vi "Sistema_Aquisicao_queued.vi"() -> ()   [LabVIEW 2012]
uses:
  Global_Telescopio.vi
panel:
  out "respQ":refnum<queue>
  out "cmdQ":refnum<queue>
  out "error out":errorcluster
  out "ultimo valor 2":dbl format="%#_9g"
  out "ultimo valor":dbl format="%#_9g"
  out "ultimo comando":dbl
  in  "Case Constant\n(See Context Help)":bool=TRUE
  out "O Recebido":bool
  out "TimeoutAq":u32
  out "concatenated string":string
  out "Maq Satus":i32
  out "TX":string
  out "Data rx Aquisição":string
  # "2"
  # "R -->Registra Centragem\nS -->Status\nO -->OffSet\nF ---> Foco"
  # "3"
  # "4"
  # "5"
  # "!"
  # "!"
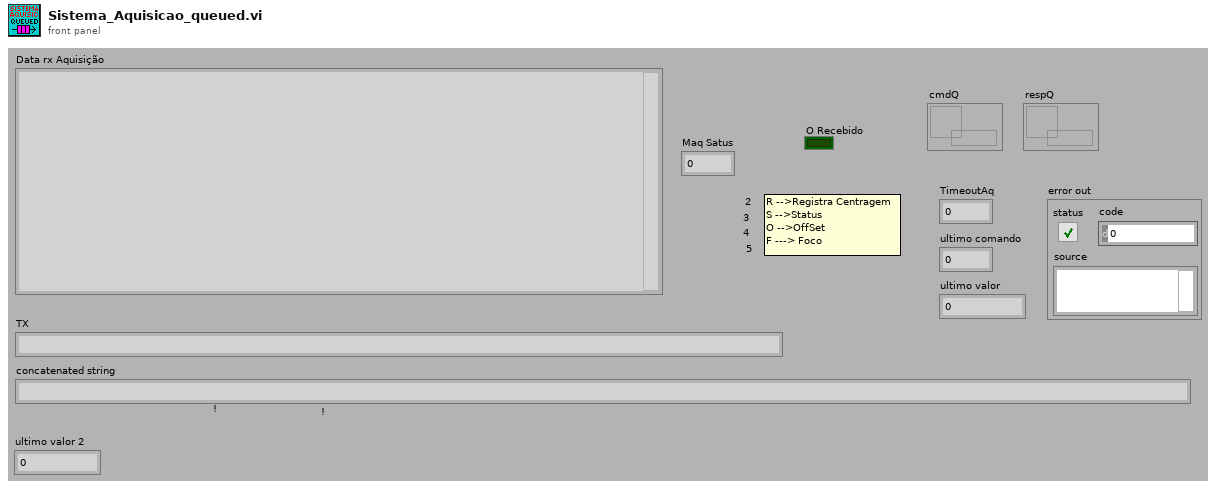
[diagram p1: front panel]
types:
  T1 = enum16{"open", "open or create", "create or replace", "create"}
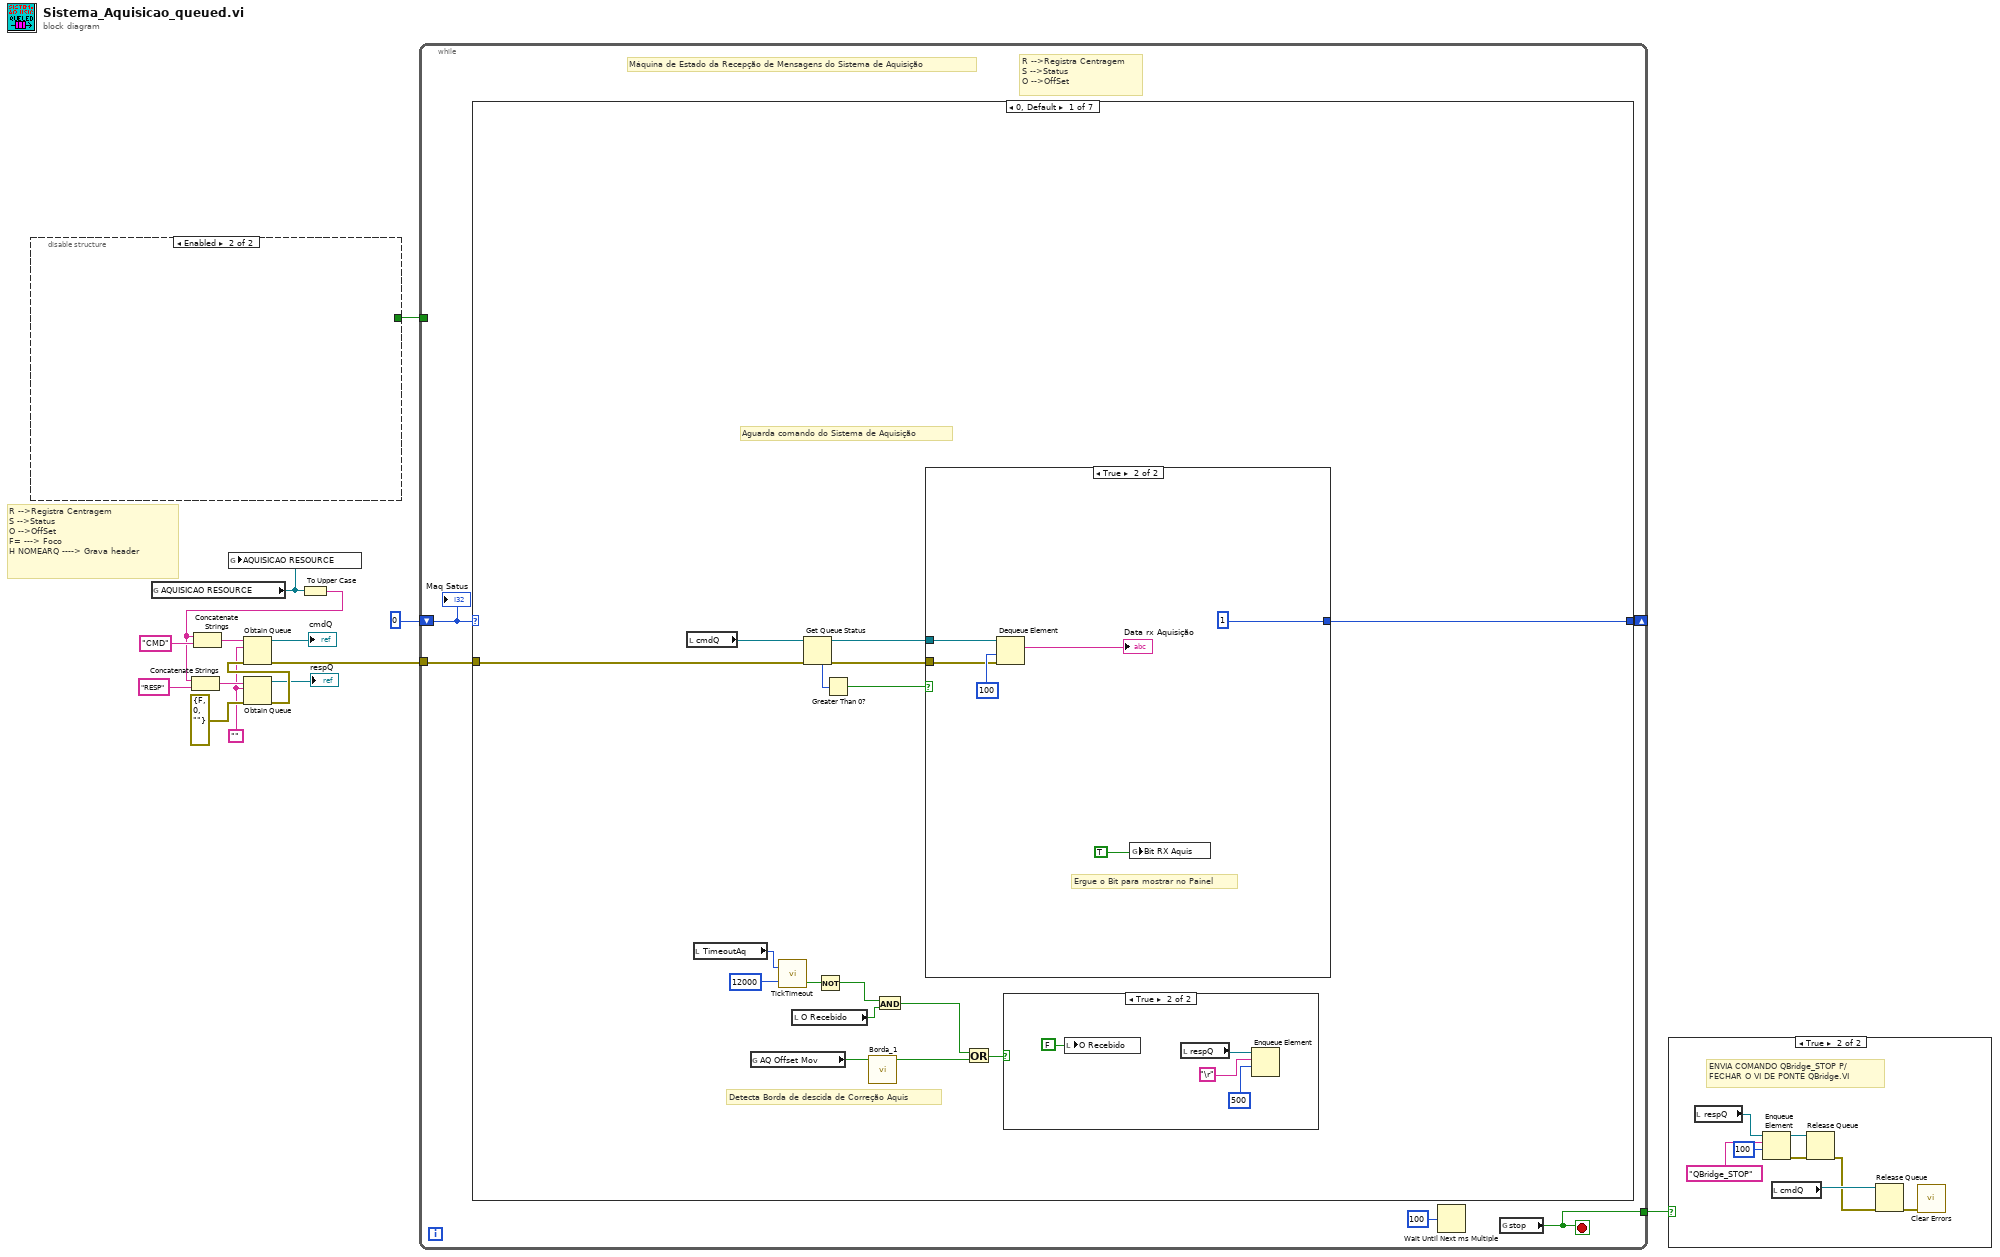
[diagram p0: block diagram]
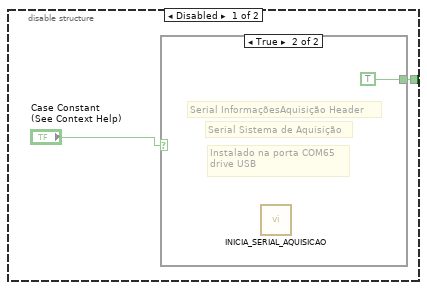
[diagram p3: hidden frame]
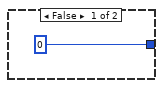
[diagram p6: hidden frame]
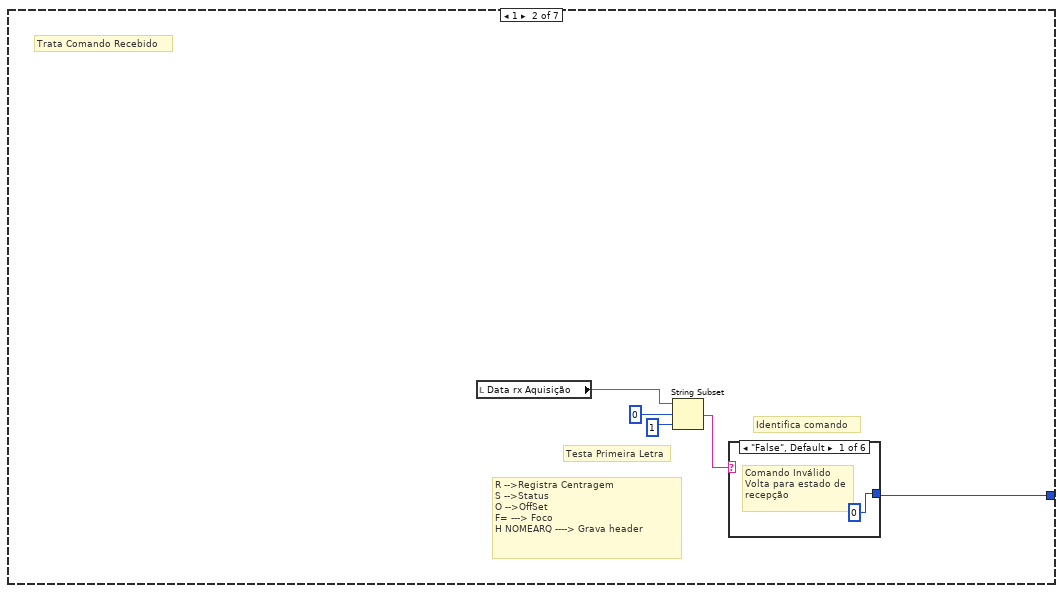
[diagram p7: hidden frame]
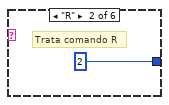
[diagram p8: hidden frame]
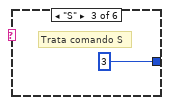
[diagram p9: hidden frame]
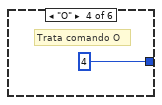
[diagram p10: hidden frame]
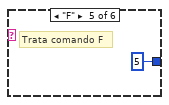
[diagram p11: hidden frame]
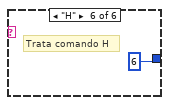
[diagram p12: hidden frame]
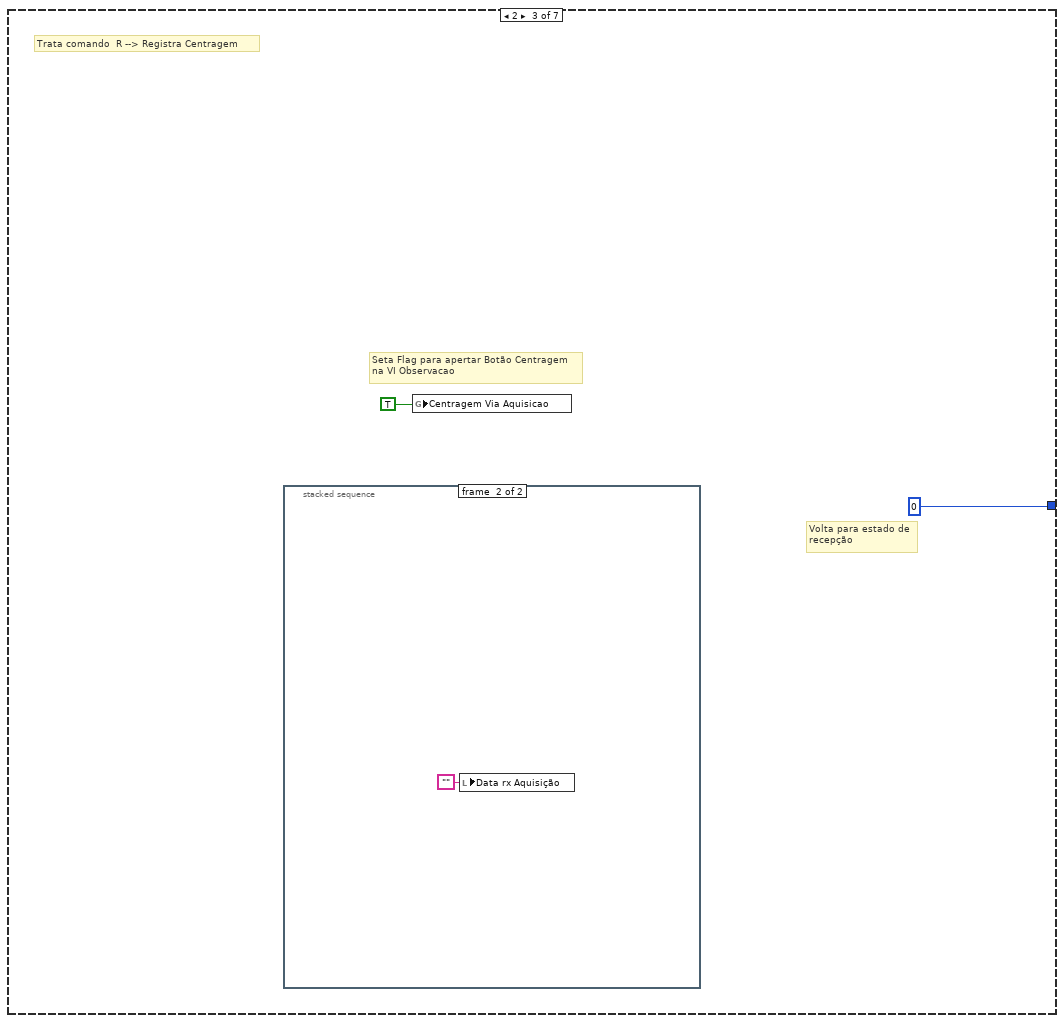
[diagram p13: hidden frame]
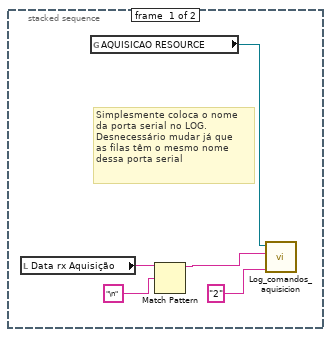
[diagram p14: hidden frame]
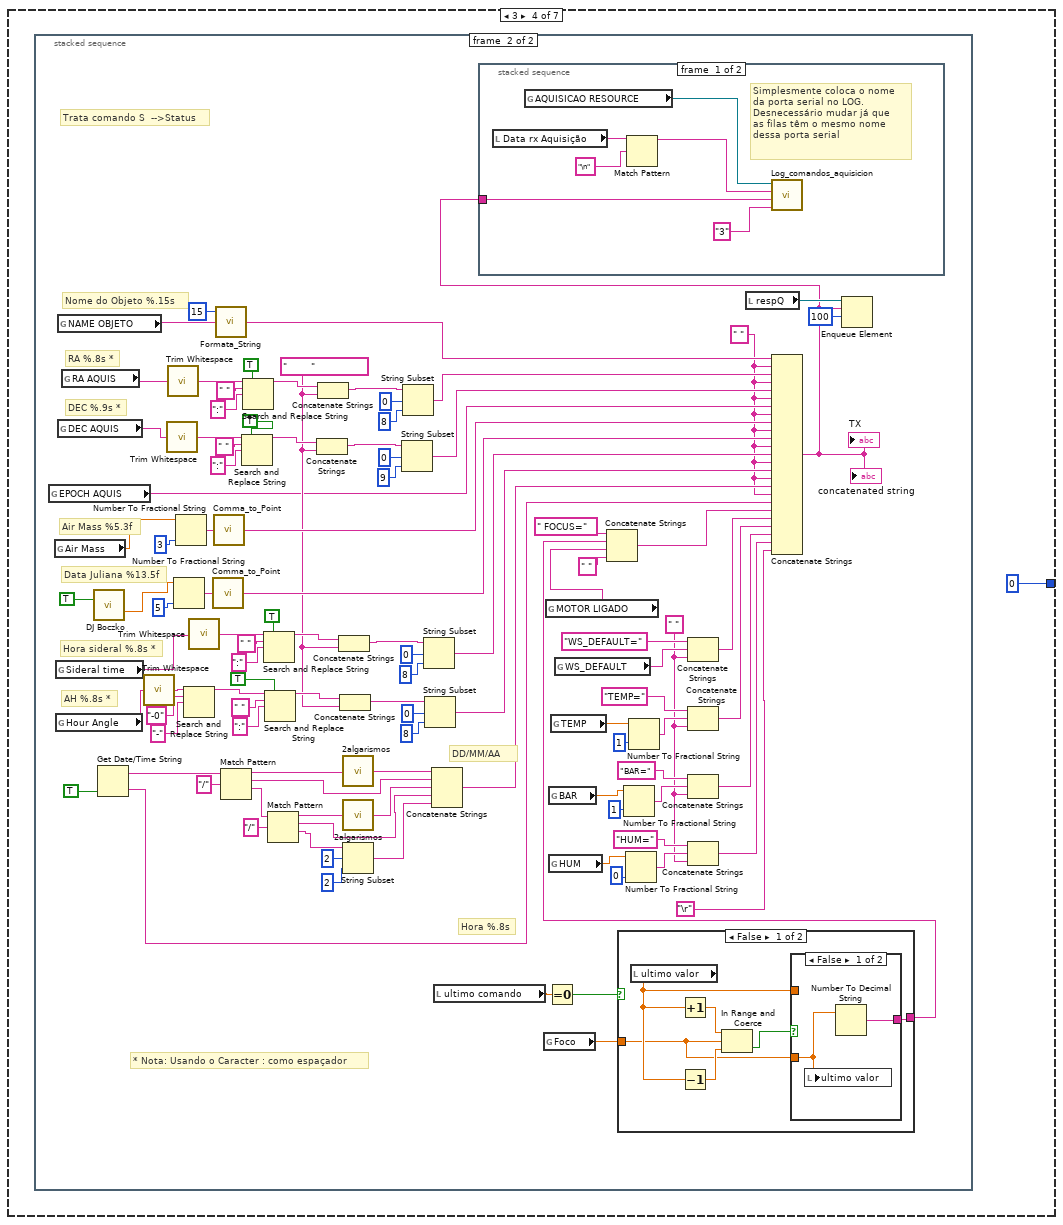
[diagram p15: hidden frame]
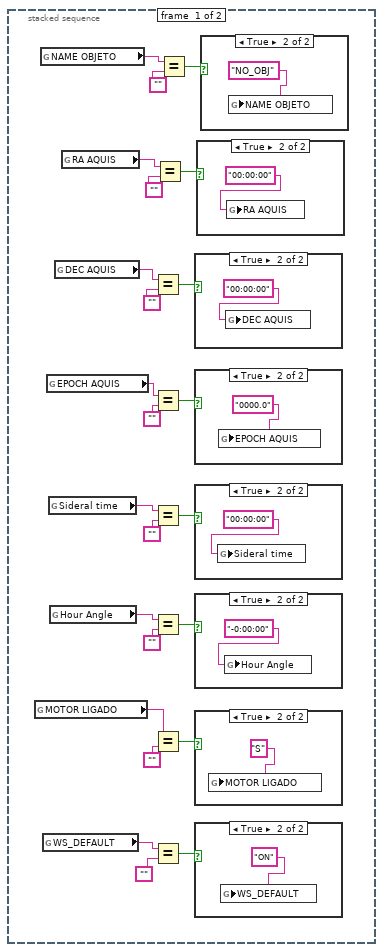
[diagram p16: hidden frame]
diagram:
  w5 = ""
  # "R -->Registra Centragem\nS -->Status\nO -->OffSet\nF= ---> Foco\nH NOMEARQ ----> Grava header"
  n1 = disable-structure shown="Enabled" {
    disable-tunnel: [w16 _] -> w14
    frame Disabled {
      n2 = case shown="True" "Case Constant\n(See Context Help)" {
        tunnel: [_ TRUE] -> w16
        frame False {
        }
        frame True {
          # "Instalado na porta COM65\ndrive USB"
          # "Serial Sistema de Aquisição"
          # "Serial InformaçõesAquisição Header"
          n3 = call "INICIA_SERIAL_AQUISICAO.vi"() -> ()  [unwired: 1 in]
        }
      }
    }
    frame Enabled {
    }
  }
  n4 = global read "Global_Telescopio.vi" "AQUISICAO RESOURCE"() -> (w3:refnum<visa-resource-name>)
  n5 = global write "Global_Telescopio.vi" "AQUISICAO RESOURCE"(w3) -> ()
  n6 = To Upper Case(1:w3) -> (0:w2:string)
  n7 = Concatenate Strings(w2, "RESP" ("string")) -> (w11:string)
  n8 = Concatenate Strings(w2, "CMD" ("string")) -> (w10:string)
  n9 = Obtain Queue(name (unnamed)=w11, element data type=w5, error in (no error)=errorcluster {"status"=FALSE, "code"=0, "source"=""}) -> (queue out=→"respQ":refnum<queue>, error out=w8:errorcluster)  [unwired: 2 in, 1 out]
  n10 = Obtain Queue(name (unnamed)=w10, element data type=w5, error in (no error)=w8) -> (queue out=→"cmdQ":refnum<queue>, error out=w4:errorcluster)  [unwired: 2 in, 1 out]
  n11 = while {
    shift-right: [w21] -> _
    shift-left: 0 -> [w22]
    tunnel: w14 -> [_]
    tunnel: w4 -> [w20]
    tunnel: [w19] -> w1
    stop <- w19 stop-if-true
    # "R -->Registra Centragem\nS -->Status\nO -->OffSet"
    # "Máquina de Estado da Recepção de Mensagens do Sistema de Aquisição"
    n12 = case shown="0, Default" w22 {
      tunnel: [w39 w51 0 0 0 0 0] -> w21
      tunnel: w20 -> [w25 _ _ _ _ _ _]
      frame 0, Default {
        # "Detecta Borda de descida de Correção Aquis"
        # "Aguarda comando do Sistema de Aquisição"
        n13 = local read "cmdQ"() -> (w24:refnum<queue>)
        n14 = local read "TimeoutAq"() -> (w32:u32)
        n15 = global read "Global_Telescopio.vi" "AQ Offset Mov"() -> (w37:bool)
        n16 = call "TickTimeout.vi"("msInicial"=w32, "msTimeout"=u32 12000) -> ("Timeout"=w33:bool)  [unwired: 2 out]
        n17 = local read "O Recebido"() -> (w35:bool)
        n18 = Get Queue Status(queue=w24, error in (no error)=w25) -> (queue out=w26:refnum<queue>, error out=w27:errorcluster, # elements in queue=w29:i32)  [unwired: 1 in, 5 out]
        n19 = Not(x=w33) -> (.not. x?=w31:bool)
        n20 = Greater Than 0?(x=w29) -> (x > 0?=w28:bool)
        n21 = call "Borda_1.vi"("Entrada"=w37) -> ("Boolean"=w38:bool)  [unwired: 4 in]
        n22 = And(x=w31, y=w35) -> (x .and. y?=w30:bool)
        n23 = case shown="True" w28 {
          tunnel: [0 1] -> w39
          tunnel: w27 -> [_ w46]
          tunnel: w26 -> [_ w47]
          frame False {
          }
          frame True {
            # "Ergue o Bit para mostrar no Painel"
            n24 = Dequeue Element(queue=w47, timeout in ms (-1)=100, error in (no error)=w46) -> (element=→"Data rx Aquisição":string)  [unwired: 3 out]
            n25 = global write "Global_Telescopio.vi" "Bit RX Aquis"(TRUE) -> ()
          }
        }
        n26 = Or(x=w30, y=w38) -> (x .or. y?=w36:bool)
        n27 = case shown="True" w36 {
          frame False {
          }
          frame True {
            n28 = local write "O Recebido"(FALSE ("O Recebido")) -> ()
            n29 = local read "respQ"() -> (w42:refnum<queue>)
            n30 = Enqueue Element(queue=w42, element="\r", timeout in ms (-1)=500) -> ()  [unwired: 1 in, 3 out]
          }
        }
      }
      frame 1 {
        # "R -->Registra Centragem\nS -->Status\nO -->OffSet\nF= ---> Foco\nH NOMEARQ ----> Grava header"
        # "Testa Primeira Letra"
        # "Identifica comando"
        # "Trata Comando Recebido"
        n31 = local read "Data rx Aquisição"() -> (w52:string)
        n32 = String Subset(string=w52, offset (0)=0, length (rest)=1 ("length (rest)")) -> (substring=w55:string)
        n33 = case shown="\"False\", Default" w55 {
          tunnel: [0 2 3 4 5 6] -> w51
          frame "False", Default {
            # "Comando Inválido\nVolta para estado de\nrecepção"
          }
          frame "R" {
            # "Trata comando R"
          }
          frame "S" {
            # "Trata comando S"
          }
          frame "O" {
            # "Trata comando O"
          }
          frame "F" {
            # "Trata comando F"
          }
          frame "H" {
            # "Trata comando H"
          }
        }
      }
      frame 2 {
        # "Seta Flag para apertar Botão Centragem\nna VI Observacao"
        # "Trata comando  R --> Registra Centragem"
        # "Volta para estado de\nrecepção"
        n34 = stacked-sequence {
          frame #0 {
            # "Simplesmente coloca o nome\nda porta serial no LOG.\nDesnecessário mudar já que \nas filas têm o mesmo nome\ndessa porta serial"
            n35 = local read "Data rx Aquisição"() -> (w65:string)
            n36 = global read "Global_Telescopio.vi" "AQUISICAO RESOURCE"() -> (w68:refnum<visa-resource-name>)
            n37 = Match Pattern(string=w65, regular expression="\n") -> (before substring=w64:string)  [unwired: 1 in, 3 out]
            n38 = call "Log_comandos_aquisicion.vi"("Estado"="2", "string de comando"=w64, "Porta"=w68) -> ()  [unwired: 9 in]
          }
          frame #1 {
            n39 = local write "Data rx Aquisição"("") -> ()
          }
        }
        n40 = global write "Global_Telescopio.vi" "Centragem Via Aquisicao"(TRUE ("Comunicaçao ok guider")) -> ()
      }
      frame 3 {
        n41 = stacked-sequence {
          frame #0 {
            n42 = global read "Global_Telescopio.vi" "MOTOR LIGADO"() -> (w91:string)
            n43 = global read "Global_Telescopio.vi" "NAME OBJETO"() -> (w72:string)
            n44 = global read "Global_Telescopio.vi" "WS_DEFAULT"() -> (w93:string)
            n45 = global read "Global_Telescopio.vi" "EPOCH AQUIS"() -> (w81:string)
            n46 = global read "Global_Telescopio.vi" "Sideral time"() -> (w83:string)
            n47 = global read "Global_Telescopio.vi" "Hour Angle"() -> (w88:string)
            n48 = global read "Global_Telescopio.vi" "DEC AQUIS"() -> (w79:string)
            n49 = global read "Global_Telescopio.vi" "RA AQUIS"() -> (w76:string)
            n50 = Equal?(x=w79, y="") -> (x = y?=w78:bool)
            n51 = Equal?(x=w81, y="") -> (x = y?=w80:bool)
            n52 = Equal?(x=w83, y="") -> (x = y?=w82:bool)
            n53 = Equal?(x=w88, y="") -> (x = y?=w84:bool)
            n54 = Equal?(x=w91, y="") -> (x = y?=w90:bool)
            n55 = Equal?(x=w93, y="") -> (x = y?=w92:bool)
            n56 = Equal?(x=w76, y="") -> (x = y?=w74:bool)
            n57 = Equal?(x=w72, y="") -> (x = y?=w73:bool)
            n58 = case shown="True" w78 {
              frame False {
              }
              frame True {
                n59 = global write "Global_Telescopio.vi" "DEC AQUIS"("00:00:00" ("NAME OBJETO")) -> ()
              }
            }
            n60 = case shown="True" w80 {
              frame False {
              }
              frame True {
                n61 = global write "Global_Telescopio.vi" "EPOCH AQUIS"("0000.0" ("NAME OBJETO")) -> ()
              }
            }
            n62 = case shown="True" w82 {
              frame False {
              }
              frame True {
                n63 = global write "Global_Telescopio.vi" "Sideral time"("00:00:00" ("NAME OBJETO")) -> ()
              }
            }
            n64 = case shown="True" w84 {
              frame False {
              }
              frame True {
                n65 = global write "Global_Telescopio.vi" "Hour Angle"("-0:00:00" ("NAME OBJETO")) -> ()
              }
            }
            n66 = case shown="True" w90 {
              frame False {
              }
              frame True {
                n67 = global write "Global_Telescopio.vi" "MOTOR LIGADO"("S") -> ()
              }
            }
            n68 = case shown="True" w92 {
              frame False {
              }
              frame True {
                n69 = global write "Global_Telescopio.vi" "WS_DEFAULT"("ON" ("Hora a ser Procurada")) -> ()
              }
            }
            n70 = case shown="True" w74 {
              frame False {
              }
              frame True {
                n71 = global write "Global_Telescopio.vi" "RA AQUIS"("00:00:00" ("NAME OBJETO")) -> ()
              }
            }
            n72 = case shown="True" w73 {
              frame False {
              }
              frame True {
                n73 = global write "Global_Telescopio.vi" "NAME OBJETO"("NO_OBJ" ("NAME OBJETO")) -> ()
              }
            }
          }
          frame #1 {
            w111 = " " ("string")
            w165 = "        " ("string")
            w120 = " "
            # "* Nota: Usando o Caracter : como espaçador"
            # "Hora %.8s"
            # "DD/MM/AA"
            # "AH %.8s *"
            # "Hora sideral %.8s *"
            # "Data Juliana %13.5f"
            # "Air Mass %5.3f"
            # "DEC %.9s *"
            # "RA %.8s *"
            # "Nome do Objeto %.15s"
            # "Trata comando S  -->Status"
            n74 = global read "Global_Telescopio.vi" "EPOCH AQUIS"() -> (w135:string)
            n75 = global read "Global_Telescopio.vi" "Air Mass"() -> (w144:dbl)
            n76 = global read "Global_Telescopio.vi" "Sideral time"() -> (w174:string)
            n77 = global read "Global_Telescopio.vi" "Hour Angle"() -> (w136:string)
            n78 = global read "Global_Telescopio.vi" "NAME OBJETO"() -> (w143:string)
            n79 = global read "Global_Telescopio.vi" "DEC AQUIS"() -> (w191:string)
            n80 = global read "Global_Telescopio.vi" "RA AQUIS"() -> (w206:string)
            n81 = call "DJ Boczko.vi"("TRUE = Hora Local\nFALSE = UT"=TRUE ("TRUE = Hora Local\nFALSE = UT")) -> ("Dia Juliano"=w184:dbl)  [unwired: 6 in, 8 out]
            n82 = Get Date/Time String(want seconds? (F)=TRUE) -> (date string=w162:string, time string=w147:string)  [unwired: 2 in]
            n83 = call <vilib>:"Trim Whitespace.vi"("string"=w136) -> ("trimmed string"=w137:string)  [unwired: 1 in]
            n84 = call <vilib>:"Trim Whitespace.vi"("string"=w191) -> ("trimmed string"=w194:string)  [unwired: 1 in]
            n85 = call <vilib>:"Trim Whitespace.vi"("string"=w206) -> ("trimmed string"=w205:string)  [unwired: 1 in]
            n86 = Number To Fractional String(number=w184, precision (6)=i16 5) -> (F-format string=w183:string)  [unwired: 2 in]
            n87 = Number To Fractional String(number=w144, precision (6)=i16 3) -> (F-format string=w187:string)  [unwired: 2 in]
            n88 = Search and Replace String(input string=w137, search string="-0", replace string="-" ("replace string (\"\")")) -> (result string=w138:string)  [unwired: 5 in, 3 out]
            n89 = call <vilib>:"Trim Whitespace.vi"("string"=w174) -> ("trimmed string"=w177:string)  [unwired: 1 in]
            n90 = call "Comma_to_Point.vi"("Lat_A"=w183) -> ("Saída"=w182:string)
            n91 = call "Comma_to_Point.vi"("Lat_A"=w187) -> ("Saída"=w186:string)
            n92 = call "Formata_String.vi"("entrada"=w143, "Num de Caracteres"=15) -> ("saida"=w141:string)  [unwired: 3 in]
            n93 = Match Pattern(string=w162, regular expression="/") -> (before substring=w158:string, match substring=w152:string, after substring=w159:string)  [unwired: 1 in, 1 out]
            n94 = Search and Replace String(replace all?=TRUE ("replace all? (F)"), input string=w194, search string=" ", replace string=":" ("replace string (\"\")")) -> (result string=w197:string)  [unwired: 4 in, 3 out]
            n95 = Search and Replace String(replace all?=TRUE ("replace all? (F)"), input string=w205, search string=" ", replace string=":" ("replace string (\"\")")) -> (result string=w201:string)  [unwired: 4 in, 3 out]
            n96 = Search and Replace String(replace all?=TRUE ("replace all? (F)"), input string=w177, search string=" ", replace string=":" ("replace string (\"\")")) -> (result string=w180:string)  [unwired: 4 in, 3 out]
            n97 = Search and Replace String(replace all?=TRUE ("replace all? (F)"), input string=w138, search string=" ", replace string=":" ("replace string (\"\")")) -> (result string=w167:string)  [unwired: 4 in, 3 out]
            n98 = Match Pattern(string=w159, regular expression="/") -> (before substring=w157:string, match substring=w150:string, after substring=w156:string)  [unwired: 1 in, 1 out]
            n99 = Concatenate Strings(w197, w165) -> (w198:string)
            n100 = Concatenate Strings(w201, w165) -> (w200:string)
            n101 = Concatenate Strings(w180, w165) -> (w181:string)
            n102 = Concatenate Strings(w167, w165) -> (w166:string)
            n103 = call "2algarismos.vi"("entrada"=w158) -> ("saida"=w153:string)
            n104 = call "2algarismos.vi"("entrada"=w157) -> ("saida"=w151:string)
            n105 = String Subset(string=w156, offset (0)=2, length (rest)=2 ("length (rest)")) -> (substring=w149:string)
            n106 = String Subset(string=w198, offset (0)=0, length (rest)=9 ("length (rest)")) -> (substring=w190:string)
            n107 = String Subset(string=w200, offset (0)=0, length (rest)=8 ("length (rest)")) -> (substring=w199:string)
            n108 = String Subset(string=w181, offset (0)=0, length (rest)=8 ("length (rest)")) -> (substring=w172:string)
            n109 = String Subset(string=w166, offset (0)=0, length (rest)=8 ("length (rest)")) -> (substring=w164:string)
            n110 = Concatenate Strings(w153, w152, w151, w150, w149) -> (w148:string)
            n111 = local read "ultimo comando"() -> (w134:dbl)
            n112 = global read "Global_Telescopio.vi" "Foco"() -> (w129:dbl)
            n113 = global read "Global_Telescopio.vi" "MOTOR LIGADO"() -> (w128:string)
            n114 = Equal To 0?(x=w134) -> (x = 0?=w133:bool)
            n115 = global read "Global_Telescopio.vi" "BAR"() -> (w122:dbl)
            n116 = global read "Global_Telescopio.vi" "HUM"() -> (w121:dbl)
            n117 = global read "Global_Telescopio.vi" "TEMP"() -> (w126:dbl)
            n118 = global read "Global_Telescopio.vi" "WS_DEFAULT"() -> (w118:string)
            n119 = case shown="False" w133 {
              tunnel: [w217 w227] -> w132
              tunnel: w129 -> [w216 w226]
              frame False {
                n120 = local read "ultimo valor"() -> (w218:dbl)
                n121 = Increment(x=w218) -> (x+1=w220:dbl)
                n122 = Decrement(x=w218) -> (x-1=w219:dbl)
                n123 = In Range and Coerce(upper limit=w220, x=w216, lower limit=w219) -> (In Range?=w221:bool)  [unwired: 1 out]
                n124 = case shown="False" w221 {
                  tunnel: w218 -> [_ w225]
                  tunnel: [w223 w224] -> w217
                  tunnel: w216 -> [w222 _]
                  frame False {
                    n125 = local write "ultimo valor"(w222) -> ()
                    n126 = Number To Decimal String(number=w222) -> (decimal integer string=w223:string)  [unwired: 1 in]
                  }
                  frame True {
                    n127 = Number To Decimal String(number=w225) -> (decimal integer string=w224:string)  [unwired: 1 in]
                  }
                }
              }
              frame True {
                n128 = Number To Decimal String(number=w226) -> (decimal integer string=w227:string)  [unwired: 1 in]
                "ultimo valor" <- w226
              }
            }
            n129 = Concatenate Strings(" FOCUS=" ("string"), w132, w128, " " ("string")) -> (w130:string)
            n130 = Number To Fractional String(number=w122, precision (6)=i16 1) -> (F-format string=w113:string)  [unwired: 2 in]
            n131 = Number To Fractional String(number=w121, precision (6)=i16 0) -> (F-format string=w112:string)  [unwired: 2 in]
            n132 = Number To Fractional String(number=w126, precision (6)=i16 1) -> (F-format string=w115:string)  [unwired: 2 in]
            n133 = Concatenate Strings("WS_DEFAULT=" ("string"), w118, w111) -> (w110:string)
            n134 = Concatenate Strings("TEMP=" ("string"), w115, w111) -> (w109:string)
            n135 = Concatenate Strings("BAR=" ("string"), w113, w111) -> (w108:string)
            n136 = Concatenate Strings("HUM=" ("string"), w112, w111) -> (w107:string)
            n137 = local read "respQ"() -> (w105:refnum<queue>)
            n138 = Concatenate Strings(w141, w120, w199, w120, w190, w120, w135, w120, w186, w120, w182, w120, w172, w120, w164, w120, w148, w120, w147, w130, w110, w109, w108, w107, "\r") -> (w104:string)
            "TX" <- w104
            "concatenated string" <- w104
            n139 = stacked-sequence {
              tunnel: w104 -> [w212 _]
              frame #0 {
                # "Simplesmente coloca o nome\nda porta serial no LOG.\nDesnecessário mudar já que \nas filas têm o mesmo nome\ndessa porta serial"
                n140 = local read "Data rx Aquisição"() -> (w211:string)
                n141 = global read "Global_Telescopio.vi" "AQUISICAO RESOURCE"() -> (w214:refnum<visa-resource-name>)
                n142 = Match Pattern(string=w211, regular expression="\n") -> (before substring=w209:string)  [unwired: 1 in, 3 out]
                n143 = call "Log_comandos_aquisicion.vi"("Estado"="3", "string de Resposta"=w212, "string de comando"=w209, "Porta"=w214) -> ()  [unwired: 8 in]
              }
              frame #1 {
                n144 = local write "Data rx Aquisição"("") -> ()
              }
            }
            n145 = Enqueue Element(queue=w105, element=w104, timeout in ms (-1)=100) -> ()  [unwired: 1 in, 3 out]
          }
        }
      }
      frame 4 {
        # "Trata comando O  -->OffSet"
        n146 = local read "Data rx Aquisição"() -> (w230:string)
        n147 = String Subset(string=w230, offset (0)=2, length (rest)=1 ("length (rest)")) -> (substring=w239:string)
        n148 = String Subset(string=w230, offset (0)=3, length (rest)=4 ("length (rest)")) -> (substring=w246:string)
        n149 = String Subset(string=w230, offset (0)=8, length (rest)=1 ("length (rest)")) -> (substring=w238:string)
        n150 = String Subset(string=w230, offset (0)=1, length (rest)=1 ("length (rest)")) -> (substring=w232:string)
        n151 = String Subset(string=w230, offset (0)=9, length (rest)=4 ("length (rest)")) -> (substring=w245:string)
        n152 = Fract/Exp String To Number(use system decimal point (T)=FALSE, string=w246) -> (number=w235:dbl)  [unwired: 2 in, 1 out]
        n153 = Fract/Exp String To Number(use system decimal point (T)=FALSE, string=w245) -> (number=w233:dbl)  [unwired: 2 in, 1 out]
        n154 = case shown="\"N\"" w239 {
          tunnel: [0.0 ("PreciseOffsetDEC 2") 1.0 ("PreciseOffsetDEC 2") -1.0 ("PreciseOffsetDEC 2")] -> w236
          frame " ", Default {
          }
          frame "N" {
          }
          frame "S" {
          }
        }
        n155 = case shown="\"E\"" w238 {
          tunnel: [0.0 ("PreciseOffsetDEC 2") 1.0 ("PreciseOffsetDEC 2") -1.0 ("PreciseOffsetDEC 2")] -> w234
          frame " ", Default {
          }
          frame "W" {
          }
          frame "E" {
          }
        }
        n156 = call "Salva_comando_Apend.vi"("String"=w230, "file name p/ exell"="C:\\TCS\\LOG\\Comando_O_Aquisicao.txt") -> ()  [unwired: 4 in]
        n157 = Multiply(x=w236, y=w234) -> (x*y=w240:dbl)
        n158 = Equal To 0?(x=w240) -> (x = 0?=w237:bool)
        n159 = case shown="True" w237 {
          tunnel: w236 -> [w273 _]
          tunnel: w235 -> [w272 _]
          tunnel: w234 -> [w271 _]
          tunnel: w233 -> [w270 _]
          tunnel: w232 -> [w268 _]
          tunnel: [TRUE ("Correção Aquis") FALSE ("Correção Aquis")] -> w231
          tunnel: ["" ""] -> w228
          frame False {
            n160 = Multiply(x=w273, y=w272) -> (x*y=w265:dbl)
            n161 = Multiply(x=w271, y=w270) -> (x*y=w269:dbl)
            n162 = case shown="\"1\"" w268 {
              tunnel: [1.0 ("PreciseOffsetDEC 2") w275] -> w267
              frame "0", Default {
              }
              frame "1" {
                n163 = global read "Global_Telescopio.vi" "delta_now"() -> (w276:dbl)
                n164 = Cosine(x=w276) -> (cos(x)=w277:dbl)
                n165 = Absolute Value(x=w277) -> (abs(x)=w275:dbl)
              }
            }
            n166 = Divide(x=w269, y=w267) -> (x/y=w266:dbl)
            n167 = global write "Global_Telescopio.vi" "aquis_asc"(w266) -> ()
            n168 = global write "Global_Telescopio.vi" "aquis_dec"(w265) -> ()
            n169 = call "TickTimeout.vi"() -> ("msTick"=→"TimeoutAq":u32)  [unwired: 2 in, 2 out]
          }
          frame True {
          }
        }
        "O Recebido" <- w231
        n170 = stacked-sequence {
          tunnel: w228 -> [_ w261]
          frame #0 {
            n171 = local read "Data rx Aquisição"() -> (w257:string)
            n172 = global read "Global_Telescopio.vi" "AQUISICAO RESOURCE"() -> (w260:refnum<visa-resource-name>)
            n173 = Match Pattern(string=w257, regular expression="\n") -> (before substring=w256:string)  [unwired: 1 in, 3 out]
            n174 = call "Log_comandos_aquisicion.vi"("Estado"="4", "string de comando"=w256, "Porta"=w260) -> ()  [unwired: 9 in]
          }
          frame #1 {
            n175 = local write "Data rx Aquisição"(w261) -> ()
          }
        }
        n176 = global write "Global_Telescopio.vi" "Correção Aquis"(w231) -> ()
      }
      frame 5 {
        # "Trata comando F ---> Trata o comando de foco vindo do computador de aquisição"
        n177 = local read "Data rx Aquisição"() -> (w294:string)
        n178 = Match Pattern(string=w294, regular expression="=") -> (after substring=w292:string)  [unwired: 1 in, 3 out]
        n179 = Fract/Exp String To Number(string=w292) -> (number=w288:dbl)  [unwired: 3 in, 1 out]
        n180 = In Range and Coerce(upper limit=2012.0, x=w288, lower limit=1.0) -> (In Range?=w289:bool)  [unwired: 1 out]
        n181 = case shown="True" w289 {
          tunnel: w288 -> [_ w304]
          tunnel: ["" ""] -> w286
          frame False {
          }
          frame True {
            n182 = case shown="True" TRUE {
              tunnel: ["stop" ("Comando") "go" ("Comando")] -> w303
              frame False {
              }
              frame True {
                n183 = call "TX focus FOCO.vi"("Comando"="def", "Setpoint"=20.0) -> ()  [unwired: 11 in, 3 out]
              }
            }
            n184 = call "TX focus FOCO.vi"("Comando"=w303, "Setpoint"=w304) -> ()  [unwired: 11 in, 3 out]
            "ultimo comando" <- w304
          }
        }
        n185 = stacked-sequence {
          tunnel: w286 -> [_ w300]
          frame #0 {
            n186 = local read "Data rx Aquisição"() -> (w296:string)
            n187 = global read "Global_Telescopio.vi" "AQUISICAO RESOURCE"() -> (w299:refnum<visa-resource-name>)
            n188 = Match Pattern(string=w296, regular expression="\n") -> (before substring=w295:string)  [unwired: 1 in, 3 out]
            n189 = call "Log_comandos_aquisicion.vi"("Estado"="5", "string de comando"=w295, "Porta"=w299) -> ()  [unwired: 9 in]
          }
          frame #1 {
            n190 = local write "Data rx Aquisição"(w300) -> ()
          }
        }
      }
      frame 6 {
        w334 = " " ("string")
        w388 = "        " ("string")
        w343 = " "
        # "PARECE QUE O HEADER É GRAVADO\nEM ARQUIVO AO INVÉS DE SER\nENVIADO PELA PORTA SERIAL. >>>?"
        # "ANTES DE INTRODUZIR FILAS\nESTA ESTRUTURA DISABLE JÁ\nESTAVA PRESENTE NO CÓDIGO"
        # "file name"
        # "* Nota: Usando o Caracter : como espaçador"
        # "Hora %.8s"
        # "DD/MM/AA"
        # "AH %.8s *"
        # "Hora sideral %.8s *"
        # "Data Juliana %13.5f"
        # "Air Mass %5.3f"
        # "DEC %.9s *"
        # "RA %.8s *"
        # "Nome do Objeto %.15s"
        # "Trata comando H NOMEARQ ---> Grava Header"
        n191 = global read "Global_Telescopio.vi" "EPOCH AQUIS"() -> (w358:string)
        n192 = global read "Global_Telescopio.vi" "Air Mass"() -> (w367:dbl)
        n193 = global read "Global_Telescopio.vi" "Sideral time"() -> (w397:string)
        n194 = global read "Global_Telescopio.vi" "Hour Angle"() -> (w359:string)
        n195 = global read "Global_Telescopio.vi" "NAME OBJETO"() -> (w366:string)
        n196 = global read "Global_Telescopio.vi" "DEC AQUIS"() -> (w414:string)
        n197 = global read "Global_Telescopio.vi" "RA AQUIS"() -> (w429:string)
        n198 = call "DJ Boczko.vi"("TRUE = Hora Local\nFALSE = UT"=TRUE ("TRUE = Hora Local\nFALSE = UT")) -> ("Dia Juliano"=w407:dbl)  [unwired: 6 in, 8 out]
        n199 = Get Date/Time String(want seconds? (F)=TRUE) -> (date string=w385:string, time string=w370:string)  [unwired: 2 in]
        n200 = call <vilib>:"Trim Whitespace.vi"("string"=w359) -> ("trimmed string"=w360:string)  [unwired: 1 in]
        n201 = local read "Data rx Aquisição"() -> (w328:string)
        n202 = call <vilib>:"Trim Whitespace.vi"("string"=w414) -> ("trimmed string"=w417:string)  [unwired: 1 in]
        n203 = call <vilib>:"Trim Whitespace.vi"("string"=w429) -> ("trimmed string"=w428:string)  [unwired: 1 in]
        n204 = Number To Fractional String(number=w407, precision (6)=i16 5) -> (F-format string=w406:string)  [unwired: 2 in]
        n205 = Number To Fractional String(number=w367, precision (6)=i16 3) -> (F-format string=w410:string)  [unwired: 2 in]
        n206 = Search and Replace String(input string=w360, search string="-0", replace string="-" ("replace string (\"\")")) -> (result string=w361:string)  [unwired: 5 in, 3 out]
        n207 = call <vilib>:"Trim Whitespace.vi"("string"=w397) -> ("trimmed string"=w400:string)  [unwired: 1 in]
        n208 = Match Pattern(string=w328, regular expression="H ") -> (after substring=w313:string)  [unwired: 1 in, 3 out]
        n209 = call "Comma_to_Point.vi"("Lat_A"=w406) -> ("Saída"=w405:string)
        n210 = call "Comma_to_Point.vi"("Lat_A"=w410) -> ("Saída"=w409:string)
        n211 = call "Formata_String.vi"("entrada"=w366, "Num de Caracteres"=15) -> ("saida"=w364:string)  [unwired: 3 in]
        n212 = Match Pattern(string=w385, regular expression="/") -> (before substring=w381:string, match substring=w375:string, after substring=w382:string)  [unwired: 1 in, 1 out]
        n213 = Search and Replace String(replace all?=TRUE ("replace all? (F)"), input string=w417, search string=" ", replace string=":" ("replace string (\"\")")) -> (result string=w420:string)  [unwired: 4 in, 3 out]
        n214 = Search and Replace String(replace all?=TRUE ("replace all? (F)"), input string=w428, search string=" ", replace string=":" ("replace string (\"\")")) -> (result string=w424:string)  [unwired: 4 in, 3 out]
        n215 = Search and Replace String(replace all?=TRUE ("replace all? (F)"), input string=w400, search string=" ", replace string=":" ("replace string (\"\")")) -> (result string=w403:string)  [unwired: 4 in, 3 out]
        n216 = Search and Replace String(replace all?=TRUE ("replace all? (F)"), input string=w361, search string=" ", replace string=":" ("replace string (\"\")")) -> (result string=w390:string)  [unwired: 4 in, 3 out]
        n217 = Match Pattern(string=w382, regular expression="/") -> (before substring=w380:string, match substring=w373:string, after substring=w379:string)  [unwired: 1 in, 1 out]
        n218 = Match Pattern(string=w313, regular expression="\r\n") -> (before substring=w311:string)  [unwired: 1 in, 3 out]
        n219 = Concatenate Strings(w420, w388) -> (w421:string)
        n220 = Concatenate Strings(w424, w388) -> (w423:string)
        n221 = Concatenate Strings(w403, w388) -> (w404:string)
        n222 = Concatenate Strings(w390, w388) -> (w389:string)
        n223 = call "2algarismos.vi"("entrada"=w381) -> ("saida"=w376:string)
        n224 = call "2algarismos.vi"("entrada"=w380) -> ("saida"=w374:string)
        n225 = String Subset(string=w379, offset (0)=2, length (rest)=2 ("length (rest)")) -> (substring=w372:string)
        n226 = String Subset(string=w421, offset (0)=0, length (rest)=9 ("length (rest)")) -> (substring=w413:string)
        n227 = String Subset(string=w423, offset (0)=0, length (rest)=8 ("length (rest)")) -> (substring=w422:string)
        n228 = String Subset(string=w404, offset (0)=0, length (rest)=8 ("length (rest)")) -> (substring=w395:string)
        n229 = String Subset(string=w389, offset (0)=0, length (rest)=8 ("length (rest)")) -> (substring=w387:string)
        n230 = Concatenate Strings(w376, w375, w374, w373, w372) -> (w371:string)
        n231 = local read "ultimo comando"() -> (w357:dbl)
        n232 = global read "Global_Telescopio.vi" "Foco"() -> (w352:dbl)
        n233 = global read "Global_Telescopio.vi" "MOTOR LIGADO"() -> (w351:string)
        n234 = Equal To 0?(x=w357) -> (x = 0?=w356:bool)
        n235 = global read "Global_Telescopio.vi" "BAR"() -> (w345:dbl)
        n236 = global read "Global_Telescopio.vi" "HUM"() -> (w344:dbl)
        n237 = global read "Global_Telescopio.vi" "TEMP"() -> (w349:dbl)
        n238 = global read "Global_Telescopio.vi" "WS_DEFAULT"() -> (w341:string)
        n239 = Concatenate Strings("C:\\TCS\\LOG\\HEADER\\" ("string"), w311, ".txt" ("string")) -> (w318:string)
        n240 = case shown="False" w356 {
          tunnel: [w436 w446] -> w355
          tunnel: w352 -> [w435 w445]
          frame False {
            n241 = local read "ultimo valor 2"() -> (w437:dbl)
            n242 = Increment(x=w437) -> (x+1=w439:dbl)
            n243 = Decrement(x=w437) -> (x-1=w438:dbl)
            n244 = In Range and Coerce(upper limit=w439, x=w435, lower limit=w438) -> (In Range?=w440:bool)  [unwired: 1 out]
            n245 = case shown="False" w440 {
              tunnel: w437 -> [_ w444]
              tunnel: [w442 w443] -> w436
              tunnel: w435 -> [w441 _]
              frame False {
                n246 = local write "ultimo valor 2"(w441) -> ()
                n247 = Number To Decimal String(number=w441) -> (decimal integer string=w442:string)  [unwired: 1 in]
              }
              frame True {
                n248 = Number To Decimal String(number=w444) -> (decimal integer string=w443:string)  [unwired: 1 in]
              }
            }
          }
          frame True {
            n249 = Number To Decimal String(number=w445) -> (decimal integer string=w446:string)  [unwired: 1 in]
            "ultimo valor 2" <- w445
          }
        }
        n250 = Concatenate Strings(" FOCUS=" ("string"), w355, w351, " " ("string")) -> (w353:string)
        n251 = Number To Fractional String(number=w345, precision (6)=i16 1) -> (F-format string=w336:string)  [unwired: 2 in]
        n252 = Number To Fractional String(number=w344, precision (6)=i16 0) -> (F-format string=w335:string)  [unwired: 2 in]
        n253 = Number To Fractional String(number=w349, precision (6)=i16 1) -> (F-format string=w338:string)  [unwired: 2 in]
        n254 = String To Path(string=w318) -> (path=w316:path)
        n255 = call <vilib>:"Open_Create_Replace File.vi"("function (open:0)"=T1."open or create", "file path"=w316) -> ("error out"=w323:errorcluster, "refnum"=w326:refnum<file>)  [unwired: 6 in, 2 out]
        n256 = Concatenate Strings("WS_DEFAULT=" ("string"), w341, w334) -> (w333:string)
        n257 = Concatenate Strings("TEMP=" ("string"), w338, w334) -> (w332:string)
        n258 = Concatenate Strings("BAR=" ("string"), w336, w334) -> (w331:string)
        n259 = Concatenate Strings("HUM=" ("string"), w335, w334) -> (w330:string)
        n260 = Set File Position(refnum=w326, from (0:start)=enum16{"start", "end", "current"}."end" ("pos mode (0:2)"), error in=w323) -> (refnum out=w320:refnum<file>, error out=w319:errorcluster)  [unwired: 1 in]
        n261 = Concatenate Strings(w364, w343, w422, w343, w413, w343, w358, w343, w409, w343, w405, w343, w395, w343, w387, w343, w371, w343, w370, w353, w333, w332, w331, w330, "\r") -> (w315:string)
        n262 = disable-structure shown="Disabled" {
          disable-tunnel: w315 -> [w433 _]
          frame Disabled {
            n263 = global read "Global_Telescopio.vi" "AQUISICAO RESOURCE"() -> (w434:refnum<visa-resource-name>)
            n264 = call "TX.vi"("tx_buf"=w433, "VISA resource name"=w434) -> ()  [unwired: 1 in, 3 out]
          }
          frame Enabled {
          }
        }
        n265 = Write to Text File(file (use dialog)=w320, text=w315, error in=w319) -> (refnum out=w325:refnum<file>, error out=w324:errorcluster)  [unwired: 1 in, 1 out]
        n266 = Close File(refnum=w325, error in=w324) -> (error out=→"error out":errorcluster)  [unwired: 1 out]
      }
    }
    n267 = Wait Until Next ms Multiple(millisecond multiple=u32 100) -> ()  [unwired: 1 out]
    n268 = global read "Global_Telescopio.vi" "stop"() -> (w19:bool)
    "Maq Satus" <- w22
  }
  n269 = case shown="True" w1 {
    frame False {
    }
    frame True {
      # "ENVIA COMANDO QBridge_STOP P/\nFECHAR O VI DE PONTE QBridge.VI"
      n270 = local read "respQ"() -> (w454:refnum<queue>)
      n271 = Enqueue Element(queue=w454, element="QBridge_STOP" ("x"), timeout in ms (-1)=100) -> (queue out=w453:refnum<queue>, error out=w452:errorcluster)  [unwired: 1 in, 1 out]
      n272 = local read "cmdQ"() -> (w451:refnum<queue>)
      n273 = Release Queue(queue=w453, error in (no error)=w452) -> (error out=w450:errorcluster)  [unwired: 1 in, 2 out]
      n274 = Release Queue(queue=w451, error in (no error)=w450) -> (error out=w448:errorcluster)  [unwired: 1 in, 2 out]
      n275 = call <vilib>:"Clear Errors.vi"("error in (no error)"=w448) -> ()  [unwired: 6 in, 1 out]
    }
  }
